vi "Update Fan Status.vi"(8 "error in (no error)":errorcluster, 9 "Fan B":T1, 10 "Fan A":T1, 11 "Evaporative Cooler Controller in":refnum<class "Evaporative Cooler Controller.lvclass">) -> (0 "error out":errorcluster, 3 "Evaporative Cooler Controller out":refnum<class "Evaporative Cooler Controller.lvclass">)   [LabVIEW 2018, in "Evaporative Cooler Controller.lvlib" / "Evaporative Cooler Controller.lvclass"]
doc: "Child classes should override this method to update their display or log files with the new status of the fans."
uses:
  Evaporative Cooler Controller.lvclass
  Dual Fan/Dual Fan/Fan Info.ctl
  Dual Fan/Dual Fan/Dual Fan.lvclass
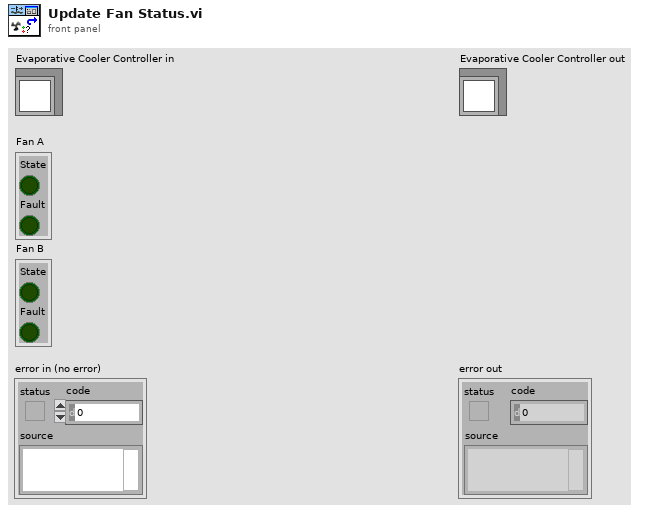
[diagram p1: front panel]
types:
  T1 = typedef "Dual Fan.lvlib/Dual Fan.lvclass/Fan Info.ctl" = cluster{"State":bool, "Fault":bool}
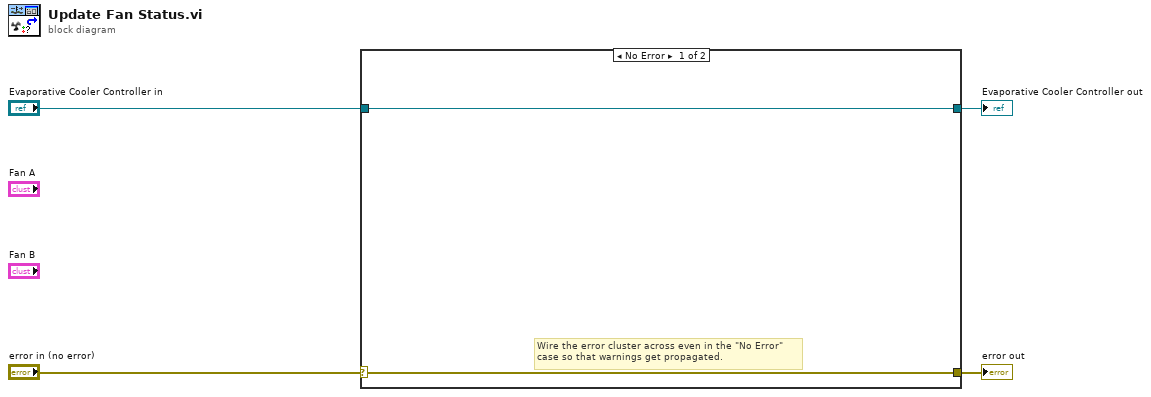
[diagram p0: block diagram]
diagram:
  n1 = case shown="No Error" "error in (no error)" {
    selector: "error in (no error)" -> [w5 w8]
    tunnel: [w5 w8] -> w3
    tunnel: [w6 w7] -> w1
    tunnel: "Evaporative Cooler Controller in" -> [w6 w7]
    frame No Error {
      # "Wire the error cluster across even in the \"No Error\"\ncase so that warnings get propagated."
    }
    frame Error {
    }
  }
  "error out" <- w3
  "Evaporative Cooler Controller out" <- w1
